vi "Pre-Process.vi"(11 "Chmmr in":refnum<class "Chmmr.lvclass">) -> (3 "Chmmr out":refnum<class "Chmmr.lvclass">)   [LabVIEW 2021, in "Chmmr.lvclass"]
uses:
  Chmmr.lvclass
  Ship/Ship.lvclass
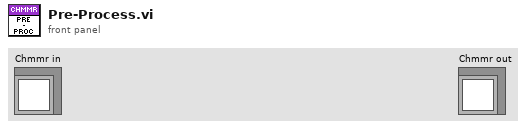
[diagram p1: front panel]
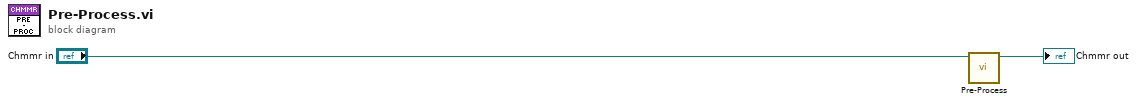
[diagram p0: block diagram]
diagram:
  n1 = call-parent "Pre-Process.vi"("Ship in"="Chmmr in") -> ("Ship out"=→"Chmmr out":refnum<class "Chmmr.lvclass">)  [unwired: 10 in]
